vi "Label Targets2.vi"(6 "Edges":cluster{"X":sgl, "Y":sgl}[](array[cluster]), 8 "Line":T1, 9 "Annotate":bool=TRUE, 10 "Results":T3 {"Score" format="%#_3g"; "Pixels"."Rectangle"."Numeric 5" format="%#_3g"; "Pixels"."Rectangle"."Numeric 3" format="%#_3g"; "Pixels"."Rectangle"."Numeric 2" format="%#_3g"; "Pixels"."Rectangle"."Numeric" format="%#_3g"; "Normalized"."Rectangle"."Numeric 5" format="%#_2g"; "Normalized"."Rectangle"."Numeric 3" format="%#_2g"; "Normalized"."Rectangle"."Numeric 2" format="%#_2g"; "Normalized"."Rectangle"."Numeric" format="%#_2g"; "Normalized"."Center"."?" format="%#_3g"; "Normalized"."Center"."?" format="%#_3g"; "Distance (ft)" format="%#_3g"}, 11 "Image in":T2) -> (3 "Image out":T2)   [LabVIEW 2016]
doc: "Draw text values near or on the particle and draws a square around the target stripes.."
uses:
  <vilib>/vision/Image Controls.llb/IMAQ Image.ctl
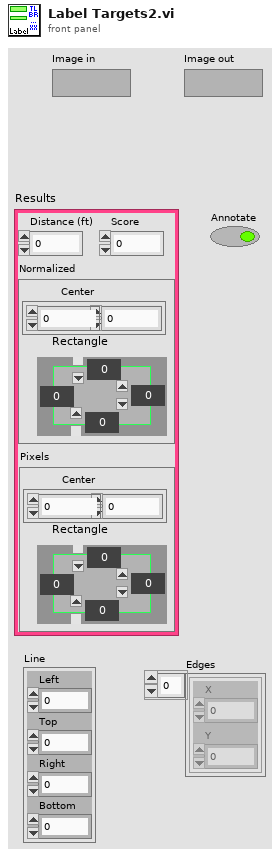
[diagram p1: front panel]
types:
  T1 = cluster{"Left":dbl, "Top":dbl, "Right":dbl, "Bottom":dbl}
  T2 = typedef "IMAQ Image.ctl" = refnum<image>
  T3 = cluster{"Distance (ft)":dbl, "Score":dbl, "Normalized":cluster{"Center":cluster{dbl, dbl}, "Rectangle":cluster{"Numeric":dbl, "Numeric 2":dbl, "Numeric 3":dbl, "Numeric 5":dbl}}, "Pixels":cluster{"Center":cluster{dbl, dbl}, "Rectangle":cluster{"Numeric":dbl, "Numeric 2":dbl, "Numeric 3":dbl, "Numeric 5":dbl}}}
  T4 = cluster{"Desired Font (Application)":enum16{"User-specified Font", "Application Font", "System Font", "Dialog Font"}, "[User-specified Font]":cluster{"Font Name":string, "Size":i16, "Strikeout?":bool, "Italic?":bool, "Underline?":bool, "Outline?":bool, "Shadow?":bool, "Bold?":bool, "Rotation Angle":dbl}, "Horizontal Alignment":i16, "Vertical Alignment":i16}
  T5 = cluster{"Left":i32, "Top":i32, "Right":i32, "Bottom":i32}
  T6 = cluster{"Center":cluster{dbl, dbl}, "Rectangle":cluster{"Numeric":dbl, "Numeric 2":dbl, "Numeric 3":dbl, "Numeric 5":dbl}}
  T7 = cluster{"Numeric":dbl, "Numeric 2":dbl, "Numeric 3":dbl, "Numeric 5":dbl}
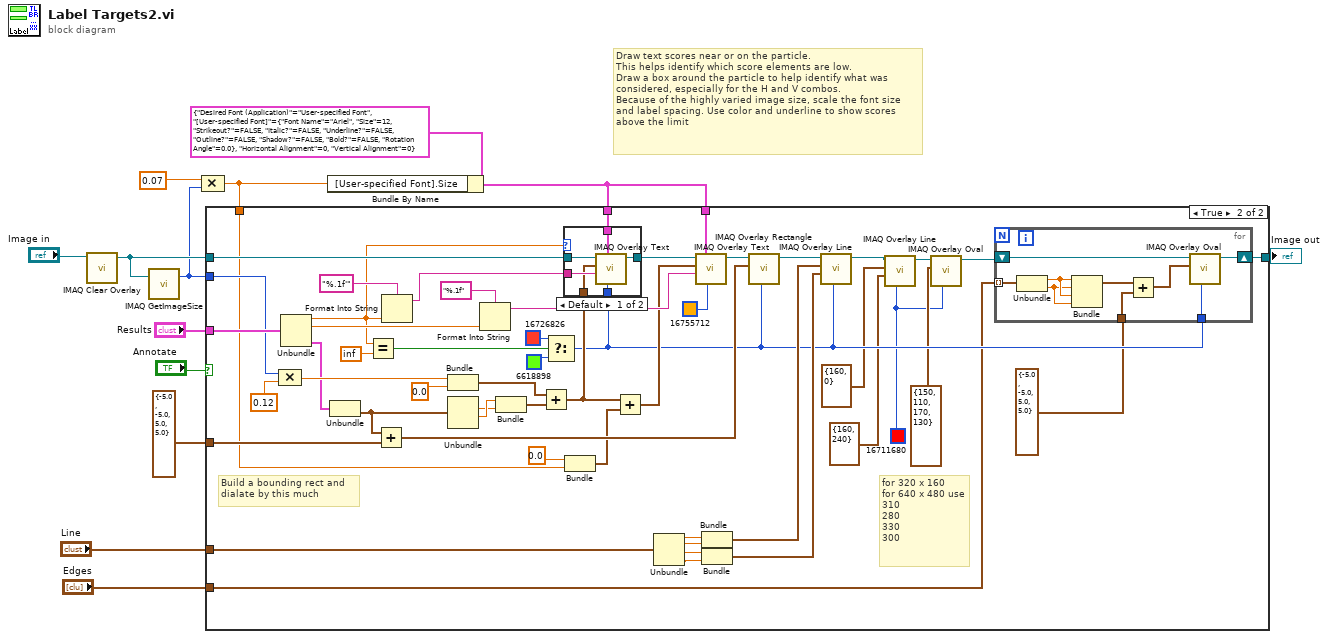
[diagram p0: block diagram]
diagram:
  # "Draw text scores near or on the particle.\nThis helps identify which score elements are low.\nDraw a box around the particle to help identify what was\nconsidered, especially for the H and V combos.\nBecause of the highly varied image size, scale the font size\nand label spacing. Use color and underline to show scores\nabove the limit"
  n1 = call "IMAQ Clear Overlay"("Image"="Image in") -> ("Image Out"=w8:T2)  [unwired: 2 in, 8 out]
  n2 = call "IMAQ GetImageSize"("Image"=w8) -> ("Y Resolution"=w7:i32)  [unwired: 3 in, 2 out]
  n3 = Compound Arithmetic op=MULTIPLY(0.07, w7) -> (w3:dbl)
  n4 = Bundle By Name(cluster=T4 {"Desired Font (Application)"=enum."User-specified Font", "[User-specified Font]"={"Font Name"="Ariel", "Size"=12, "Strikeout?"=FALSE, "Italic?"=FALSE, "Underline?"=FALSE, "Outline?"=FALSE, "Shadow?"=FALSE, "Bold?"=FALSE, "Rotation Angle"=0.0}, "Horizontal Alignment"=0, "Vertical Alignment"=0} ("Font, Size & Style"), "[User-specified Font].Size"=w3) -> (w4:T4)
  n5 = case shown="True" "Annotate" {
    tunnel: [w14 w26] -> w13
    tunnel: "Results" -> [_ w67]
    tunnel: w8 -> [w14 w66]
    tunnel: w4 -> [_ w55]
    tunnel: w7 -> [_ w65]
    tunnel: cluster{dbl, dbl, dbl, dbl} {-5.0, -5.0, 5.0, 5.0} ("output cluster") -> [_ w54]
    tunnel: w4 -> [_ w49]
    tunnel: w3 -> [_ w40]
    tunnel: "Line" -> [_ w34]
    tunnel: "Edges" -> [_ w24]
    frame False {
    }
    frame True {
      w15 = u32 16711680 ("Color")
      # "for 320 x 160\nfor 640 x 480 use\n310\n280\n330\n300"
      # "Build a bounding rect and\ndialate by this much"
      n6 = Compound Arithmetic op=MULTIPLY(w65, 0.12) -> (w58:dbl)
      n7 = Unbundle(w67) -> ("Distance (ft)"=w22:dbl, "Score"=w47:dbl, "Pixels"=w52:T6)  [unwired: 1 out]
      n8 = Unbundle(w52) -> ("Rectangle"=w53:T7)  [unwired: 1 out]
      n9 = Equal?(x=w22, y=inf) -> (x = y?=w36:bool)
      n10 = Add(x=w53, y=w54) -> (x+y=w61:cluster{dbl, dbl, dbl, dbl})
      n11 = Format Into String(format string="%.1f'", w22) -> (resulting string=w56:string)  [unwired: 2 in, 1 out]
      n12 = Bundle(w58, 0.0) -> (w60:cluster{dbl, dbl})  [unwired: 1 in]
      n13 = Unbundle(w53) -> ("Numeric 2"=w63:dbl, "Numeric 3"=w64:dbl)  [unwired: 2 out]
      n14 = Format Into String(format string="%.1f", w47) -> (resulting string=w45:string)  [unwired: 2 in, 1 out]
      n15 = Bundle("Numeric 3"=w64, "Numeric 2"=w63) -> (w62:cluster{"Numeric 3":dbl, "Numeric 2":dbl})  [unwired: 1 in]
      n16 = Add(x=w60, y=w62) -> (x+y=w44:cluster{dbl, dbl})
      n17 = Select(t=u32 16726826 ("Color"), s=w36, f=u32 6618898 ("Color")) -> (s? t:f=w25:u32)
      n18 = case shown="Default" w22 {
        tunnel: w66 -> [w73 w74]
        tunnel: w56 -> [w72 _]
        tunnel: w55 -> [w71 _]
        tunnel: [w70 w74] -> w51
        tunnel: w44 -> [w69 _]
        tunnel: w25 -> [w68 _]
        frame Default {
          n19 = call "IMAQ Overlay Text"("Text Color (black)"=w68, "Font, Size & Style"=w71, "String"=w72, "Origin"=w69, "Image"=w73) -> ("Image Out"=w70:T2)  [unwired: 5 in, 1 out]
        }
        frame 0 {
        }
      }
      n20 = Bundle(0.0, w40) -> (w43:cluster{dbl, dbl})  [unwired: 1 in]
      n21 = Add(x=w44, y=w43) -> (x+y=w41:cluster{dbl, dbl})
      n22 = Unbundle(w34) -> ("Left"=w33:dbl, "Top"=w32:dbl, "Right"=w31:dbl, "Bottom"=w30:dbl)
      n23 = call "IMAQ Overlay Text"("Text Color (black)"=u32 16755712 ("Color"), "Font, Size & Style"=w49, "String"=w45, "Origin"=w41, "Image"=w51) -> ("Image Out"=w50:T2)  [unwired: 5 in, 1 out]
      n24 = Bundle("Left"=w33, "Top"=w32) -> (w28:cluster{"Left":dbl, "Top":dbl})  [unwired: 1 in]
      n25 = Bundle("Right"=w31, "Bottom"=w30) -> (w27:cluster{"Right":dbl, "Bottom":dbl})  [unwired: 1 in]
      n26 = call "IMAQ Overlay Rectangle"("Color"=w25, "Rectangle"=w61, "Image"=w50) -> ("Image Out"=w29:T2)  [unwired: 7 in, 1 out]
      n27 = call "IMAQ Overlay Line"("Color"=w25, "End Point"=w27, "Start Point"=w28, "Image"=w29) -> ("Image Out"=w21:T2)  [unwired: 6 in, 1 out]
      n28 = call "IMAQ Overlay Line"("Color"=w15, "End Point"=cluster{"X":i32, "Y":i32} {"X"=160, "Y"=240}, "Start Point"=cluster{"X":i32, "Y":i32} {"X"=160, "Y"=0}, "Image"=w21) -> ("Image Out"=w20:T2)  [unwired: 6 in, 1 out]
      n29 = call "IMAQ Overlay Oval"("Color"=w15, "Bounding Rectangle"=T5 {"Left"=150, "Top"=110, "Right"=170, "Bottom"=130}, "Image"=w20) -> ("Image Out"=w17:T2)  [unwired: 7 in, 1 out]
      n30 = for {
        shift-right: [w82] -> w26
        shift-left: w17 -> [w83]
        tunnel: w25 -> [w81]
        tunnel: w24 -> [w79] mode=indexing
        tunnel: cluster{"X":sgl, "Y":sgl, "X":sgl, "Y":sgl} {"X"=-5.0, "Y"=-5.0, "X"=5.0, "Y"=5.0} ("output cluster") -> [w75]
        n31 = Unbundle(w79) -> ("X"=w78:sgl, "Y"=w77:sgl)
        n32 = Bundle("X"=w78, "Y"=w77, "X"=w78, "Y"=w77) -> (w76:cluster{"X":sgl, "Y":sgl, "X":sgl, "Y":sgl})  [unwired: 1 in]
        n33 = Add(x=w76, y=w75) -> (x+y=w80:cluster{"X":sgl, "Y":sgl, "X":sgl, "Y":sgl})
        n34 = call "IMAQ Overlay Oval"("Color"=w81, "Bounding Rectangle"=w80, "Image"=w83) -> ("Image Out"=w82:T2)  [unwired: 7 in, 1 out]
      }
    }
  }
  "Image out" <- w13
